vi "UDPInit.vi"(10 "port":u16) -> (2 "UDP":refnum<k16>)   [LabVIEW 2017]
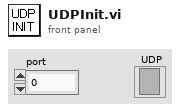
[diagram p1: front panel]
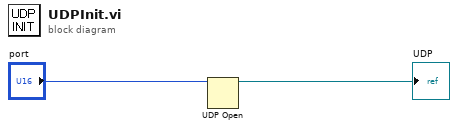
[diagram p0: block diagram]
diagram:
  n1 = UDP Open(11:"port") -> (port=→"UDP":refnum<k16>)  [unwired: 4 in, 2 out]
